vi "Set Git Application.vi"(10 "Git Application":string="git", 11 "Git Implementation in":refnum<class "Git Implementation.lvclass">) -> (3 "Git Implementation out":refnum<class "Git Implementation.lvclass">)   [LabVIEW 2017, in "Git Implementation.lvclass"]
uses:
  Git Implementation.lvclass
  Git Implementation.lvclass/Git Implementation.ctl
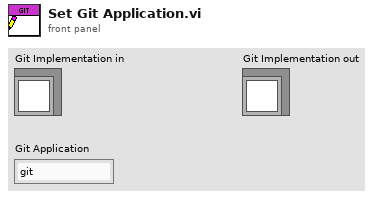
[diagram p1: front panel]
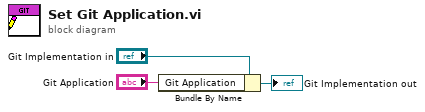
[diagram p0: block diagram]
diagram:
  n1 = Bundle By Name(cluster="Git Implementation in", "Git Application"="Git Application") -> (→"Git Implementation out":refnum<class "Git Implementation.lvclass">)
